vi "ASCII char to U8.vi"(0 "ASCII character(s)":string) -> (1 "first ASCII value (U8)":u8, 2 "byte array (U8)":u8[](array[numeric]))   [LabVIEW 2011]
doc: "ASCII Char to U8.vi converts a string of ASCII character(s) to corresponding ASCII value(s)."
panel:
  # "Purpose: This vi converts a \nstring of ASCII character(s) to \ncorresponding decimal values."
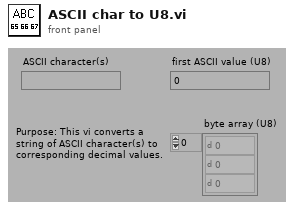
[diagram p1: front panel]
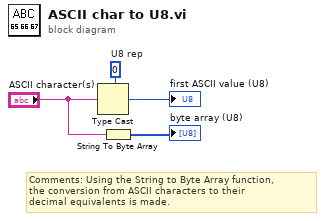
[diagram p0: block diagram]
diagram:
  w3 = u8 0  # U8 rep
  # "Comments: Using the String to Byte Array function,\nthe conversion from ASCII characters to their \ndecimal equivalents is made."
  n1 = Type Cast(type=w3, x="ASCII character(s)") -> (*(type *) &x=→"first ASCII value (U8)":u8)
  n2 = String To Byte Array(string="ASCII character(s)") -> (unsigned byte array=→"byte array (U8)":u8[])
